vi "Save TCP Ports.vi"(8 "error in":errorcluster) -> (0 "error out":errorcluster)   [LabVIEW 2024, in "Data Base.lvlib"]
uses:
  Data Base.lvlib
  Support/General Type Defs/Global Data.vi
  <vilib>/Utility/file.llb/Write Delimited Spreadsheet (string).vi
  Support/General Type Defs/General Type Definitions.lvlib
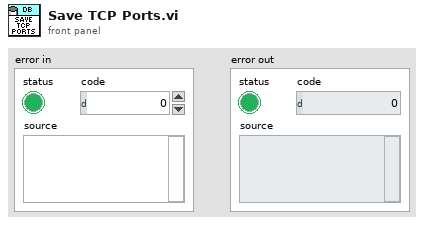
[diagram p1: front panel]
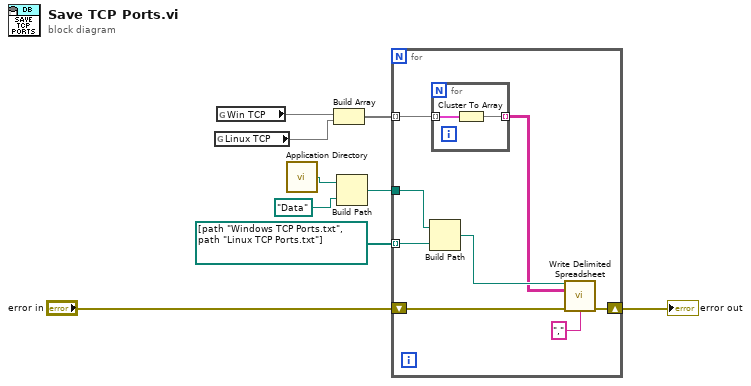
[diagram p0: block diagram]
diagram:
  n1 = global read "Global Data.vi" "Linux TCP"() -> (w3:map{string, string})
  n2 = global read "Global Data.vi" "Win TCP"() -> (w4:map{string, string})
  n3 = call <vilib>:"Application Directory.vi"() -> ("Application Directory"=w5:path)
  n4 = Build Array(w4, w3) -> (w2:map{string, string}[])
  n5 = Build Path(base path=w5, name or relative path=path "Data") -> (appended path=w7:path)
  n6 = for {
    tunnel: w7 -> [w17]
    tunnel: path[] [path "Windows TCP Ports.txt", path "Linux TCP Ports.txt"] -> [w16] mode=indexing
    shift-right: [w11] -> w1
    shift-left: "error in" -> [w14]
    tunnel: w2 -> [w15] mode=indexing
    n7 = Build Path(base path=w17, name or relative path=w16) -> (appended path=w13:path)
    n8 = for {
      tunnel: w15 -> [w19] mode=indexing
      tunnel: [w18] -> w12 mode=indexing
      n9 = Cluster To Array(cluster=w19) -> (array=w18:string[])
    }
    n10 = call-poly <vilib>:"Write Delimited Spreadsheet.vi"("file path (dialog if empty)"=w13, "2D data"=w12, "error in (no error)"=w14, "delimiter (\\t)"="," ("delimiter (\\t)")) -> ("error out"=w11:errorcluster)  [unwired: 10 in, 1 out]
  }
  "error out" <- w1
